vi "CSDB_Config.set shared variable values.vi"(3 "Type":string, 4 "AttributeName":string, 10 "Values in":string[](array[string]), 12 "InstanceNames in":string[](array[string])) -> (16 "Values out":string[](array[string]))   [LabVIEW 2014, in "CSDB_Config.lvlib"]
uses:
  CSDB_Config.lvlib
panel:
  in  "cancel":bool
  in  "Allow multiple Instances for :":string="N/A"
  out "OK":bool
  in  "done":bool
  in  "check unique":bool
  in  "apply":bool
  in  "Set Shared Variables":refnum<k21>
  in  "Table":i32[](listbox)
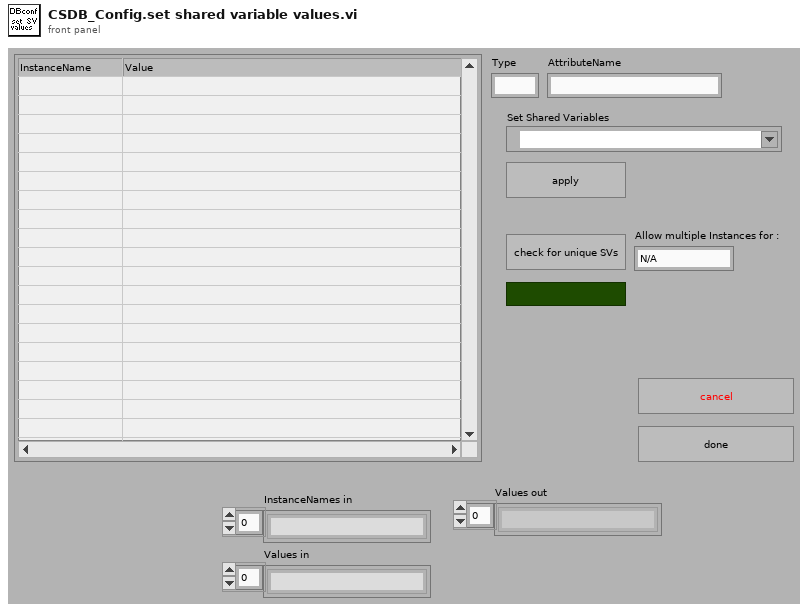
[diagram p1: front panel]
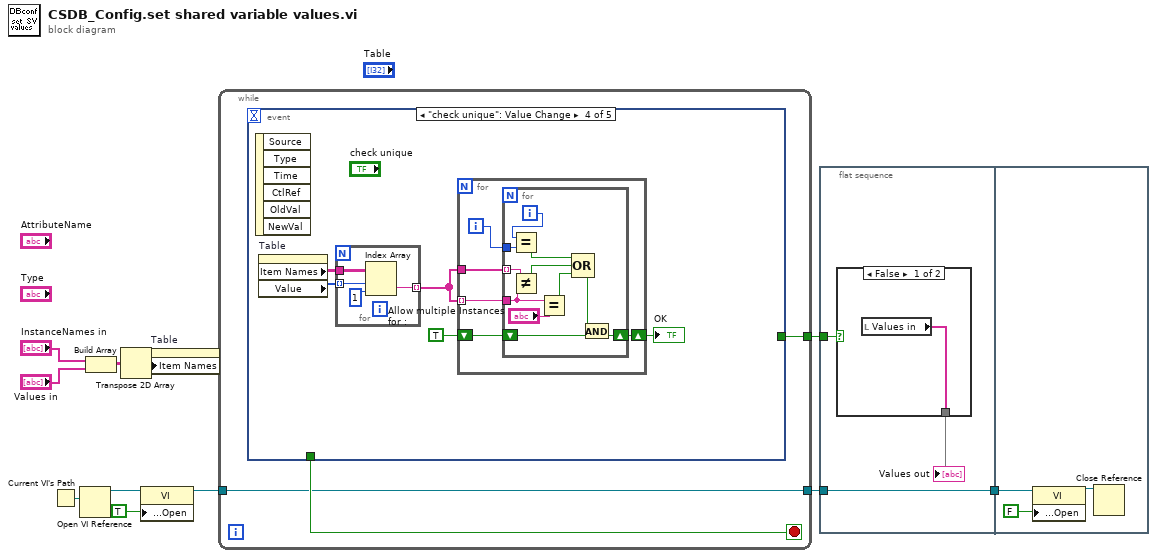
[diagram p0: block diagram]
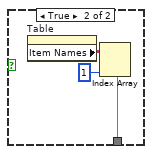
[diagram p2: hidden frame]
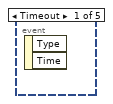
[diagram p3: hidden frame]
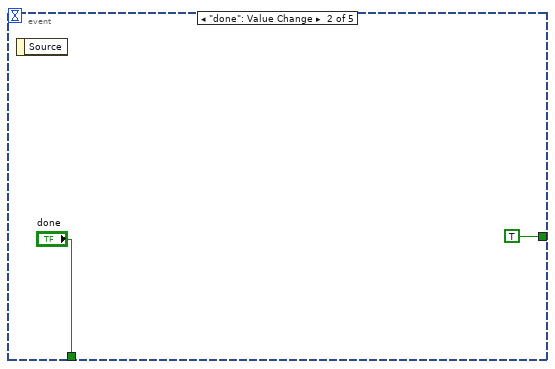
[diagram p4: hidden frame]
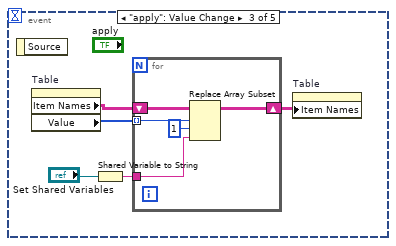
[diagram p5: hidden frame]
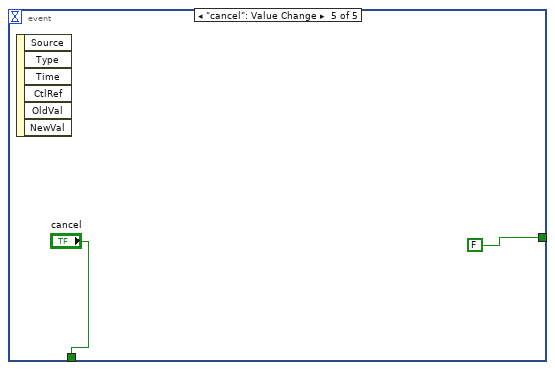
[diagram p6: hidden frame]
diagram:
  n1 = Current VI's Path() -> (path=w11:path)
  n2 = Open VI Reference(vi path=w11) -> (vi reference=w10:refnum<vi>)  [unwired: 5 in, 1 out]
  n3 = Build Array("InstanceNames in", "Values in") -> (w8:string[][])
  n4 = Transpose 2D Array(2D array=w8) -> (transposed array=w5:string[][])
  n5 = property class="VI"(reference=w10, "Front Panel Window:Open"=TRUE) -> (reference out=w4:refnum<vi>)  [unwired: 1 in, 1 out]
  n6 = property on="Table" class="MCListbox (strict)"("Item Names"=w5) -> ()  [unwired: 2 in, 2 out]
  n7 = while {
    tunnel: w4 -> [w13]
    tunnel: [w13] -> w3
    tunnel: [w12] -> w1
    stop <- w14 stop-if-true
    n8 = event shown="[3] \"check unique\": Value Change" {
      selector: _ -> [_ _ _ _ _]
      dyn-events: _ -> [_ _ _ _ _]
      timeout: _ -> [_ _ _ _ _]
      tunnel: [_ "done" _ _ "cancel"] -> w14
      tunnel: [_ TRUE _ _ FALSE] -> w12
      event Timeout {
        n9 = event-data() -> ()  [unwired: 1 in, 2 out]
      }
      event "done": Value Change {
        n10 = event-data() -> ()  [unwired: 1 in, 1 out]
      }
      event "apply": Value Change {
        n11 = event-data() -> ()  [unwired: 1 in, 1 out]
        n12 = property on="Table" class="MCListbox (strict)"() -> ("Item Names"=w18:string[][], "Value"=w20:i32[])  [unwired: 2 in, 2 out]
        n13 = Shared Variable to String(1:"Set Shared Variables") -> (0:w19:string)
        n14 = for {
          tunnel: w20 -> [w26] mode=indexing
          tunnel: w19 -> [w24]
          shift-right: [w22] -> w17
          shift-left: w18 -> [w23]
          n15 = Replace Array Subset(array=w23, new element=w24, index (row)=w26, index (col)=1 ("disabled index (col)")) -> (w22:string[][])
        }
        n16 = property on="Table" class="MCListbox (strict)"("Item Names"=w17) -> ()  [unwired: 2 in, 2 out]
      }
      event "check unique": Value Change {
        n17 = event-data() -> ()  [unwired: 1 in, 6 out]
        n18 = property on="Table" class="MCListbox (strict)"() -> ("Item Names"=w29:string[][], "Value"=w28:i32[])  [unwired: 2 in, 2 out]
        n19 = for {
          tunnel: w29 -> [w35]
          tunnel: w28 -> [w34] mode=indexing
          tunnel: [w32] -> w27 mode=indexing
          n20 = Index Array(array=w35, index (row)=w34, index (col)=1 ("disabled index (col)")) -> (element=w32:string)
        }
        n21 = for {
          tunnel: w27 -> [w39] mode=indexing
          tunnel: w27 -> [w40]
          shift-right: [w37] -> w30
          shift-left: TRUE -> [w38]
          i -> [w36]
          n22 = for {
            tunnel: w40 -> [w51] mode=indexing
            tunnel: w39 -> [w43]
            tunnel: w36 -> [w50]
            shift-right: [w46] -> w37
            shift-left: w38 -> [w45]
            i -> [w49]
            n23 = Equal?(x=w49, y=w50) -> (x = y?=w47:bool)
            n24 = Not Equal?(x=w51, y=w43) -> (x != y?=w48:bool)
            n25 = Equal?(x=w43, y="Allow multiple Instances for :") -> (x = y?=w41:bool)
            n26 = Compound Arithmetic op=OR(w47, w48, w41) -> (w44:bool)
            n27 = And(x=w44, y=w45) -> (x .and. y?=w46:bool)
          }
        }
        "OK" <- w30
      }
      event "cancel": Value Change {
        n28 = event-data() -> ()  [unwired: 1 in, 6 out]
      }
    }
  }
  n29 = flat-sequence {
    tunnel: w3 -> [w55]
    tunnel: [w55] -> w2
    tunnel: w1 -> [w54]
    tunnel: w2 -> [w61]
    frame #0 {
      n30 = case shown="False" w54 {
        tunnel: [w57 w58] -> w56
        frame False {
          n31 = local read "Values in"() -> (w57:string[])
        }
        frame True {
          n32 = property on="Table" class="MCListbox (strict)"() -> ("Item Names"=w59:string[][])  [unwired: 2 in, 2 out]
          n33 = Index Array(array=w59, index (col)=1 ("disabled index (col)")) -> (element=w58:string[])  [unwired: 1 in]
        }
      }
      "Values out" <- w56
    }
    frame #1 {
      n34 = property class="VI"(reference=w61, "Front Panel Window:Open"=FALSE) -> (reference out=w62:refnum<vi>)  [unwired: 1 in, 1 out]
      n35 = Close Reference(reference=w62) -> ()  [unwired: 1 in, 1 out]
    }
  }
